vi "open.vi"(8 "error in (no error)":errorcluster caption="错误输入（无错误）", 10 "VISA resource name":refnum<visa-resource-name> caption="VISA资源名称", 11 "Primary Productivity 输入":refnum<class "Primary Productivity.lvclass">) -> (0 "error out":errorcluster caption="错误输出", 3 "Primary Productivity 输出":refnum<class "Primary Productivity.lvclass">)   [LabVIEW 2016, in "Primary Productivity.lvclass"]
uses:
  Primary Productivity.lvclass
  Primary Productivity.lvclass/Primary Productivity.ctl
  <vilib>/Instr/_visa.llb/VISA Configure Serial Port (Instr).vi
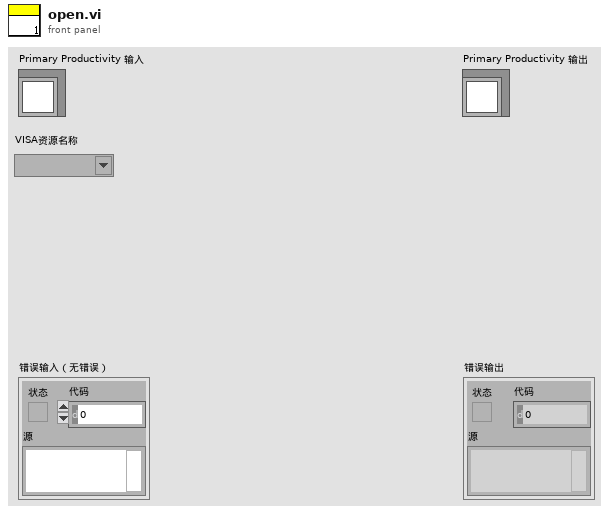
[diagram p1: front panel]
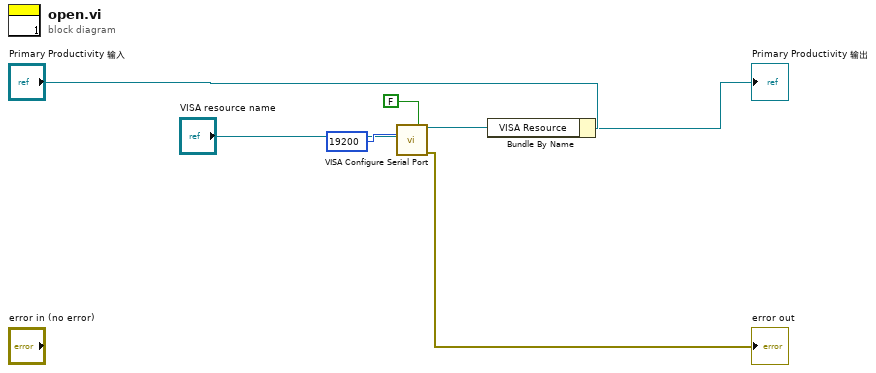
[diagram p0: block diagram]
diagram:
  n1 = call-poly "VISA Configure Serial Port"("VISA resource name"="VISA resource name", "Enable Termination\nChar (T)"=FALSE ("Enable Termination\nChar (T)"), "baud rate (9600)"=u32 19200) -> ("VISA resource name out"=w2:refnum<visa-resource-name>, "error out"=→"error out":errorcluster)  [unwired: 11 in]
  n2 = Bundle By Name(cluster="Primary Productivity 输入", "VISA Resource"=w2) -> (→"Primary Productivity 输出":refnum<class "Primary Productivity.lvclass">)
